vi "Test_StartMessageCycle_StopActor_OneOrMoreReceived.vi"(8 "error in (no error)":errorcluster, 11 "TestCase in":refnum<class "TestMessageCycle.lvclass">) -> (0 "error out":errorcluster, 3 "TestCase out":refnum<class "TestMessageCycle.lvclass">)   [LabVIEW 2017, in "TestMessageCycle.lvclass"]
uses:
  TestMessageCycle.lvclass
  Source/MessageCycle/MessageCycle.lvclass/MessageCycle.ctl
  <vilib>/ActorFramework/Message Enqueuer/Message Enqueuer.lvclass/Message Enqueuer.ctl
  <vilib>/ActorFramework/Message Enqueuer/Enqueue.vi
  Doubles/MessageCountsExecutions/MessageCountsExecutions.lvclass
  C:/Program Files (x86)/National Instruments/LabVIEW 2017/vi.lib/ActorFramework/Message/Message.lvclass
  Doubles/ActorCountsMessageCycles/ActorCountsMessageCycles.lvclass
  C:/Program Files (x86)/National Instruments/LabVIEW 2017/vi.lib/ActorFramework/Actor/Actor.lvclass
  Source/MessageCycle/MessageCycle.lvclass
  <vilib>/ActorFramework/Stop Msg/Stop Msg.lvclass
  Source/MessageCycle/Launch Deferred Timeout Notifier.vi
  <vilib>/ActorFramework/Message Priority Queue/Priority Enqueue.vi
  <vilib>/ActorFramework/Message/Message.lvclass
  <vilib>/ActorFramework/Actor/Actor.lvclass
panel:
  out "Messages Executed":u32
  out "Cyclic Messages Received":u32
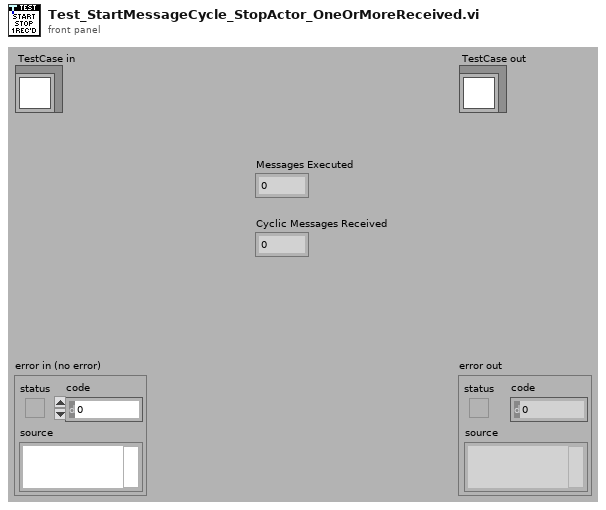
[diagram p1: front panel]
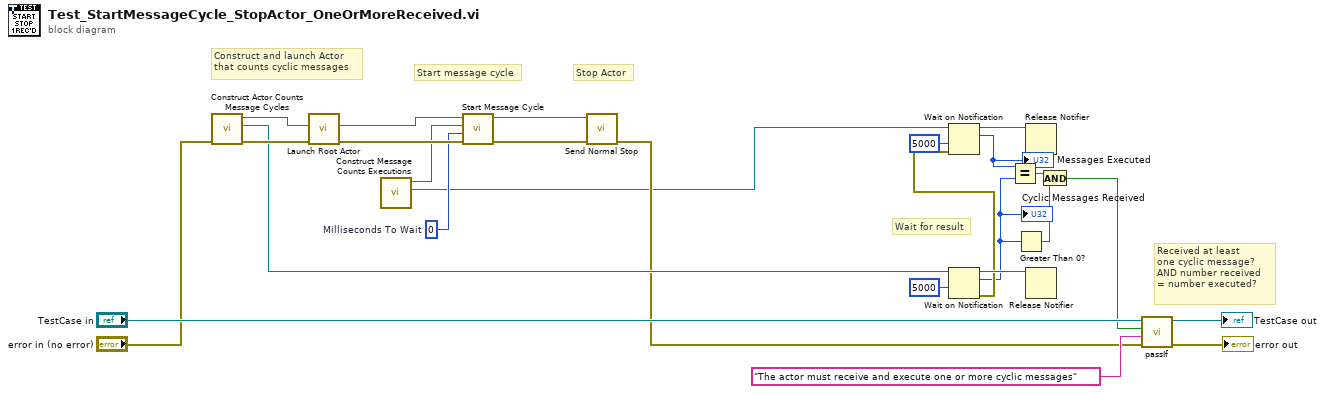
[diagram p0: block diagram]
diagram:
  w22 = 0  # Milliseconds To Wait
  # "Wait for result"
  # "Stop Actor"
  # "Start message cycle"
  # "Received at least\none cyclic message?\nAND number received\n= number executed?"
  # "Construct and launch Actor\nthat counts cyclic messages"
  n1 = call "Construct Actor Counts Message Cycles.vi"("error in (no error)"="error in (no error)") -> ("error out"=w15:errorcluster, "Final Count"=w14:refnum<notifier>, "ActorCountsMessageCycles"=w17:refnum<class "ActorCountsMessageCycles.lvclass">)  [unwired: 8 in]
  n2 = call <vilib>:"Launch Root Actor.vi"("error in (no error)"=w15, "Actor"=w17) -> ("error out"=w26:errorcluster, "Actor's Enqueuer"=w20:refnum<class "Message Enqueuer.lvclass">)  [unwired: 8 in]
  n3 = call "Construct Message Counts Executions.vi"() -> ("Message Executions"=w7:refnum<notifier>, "CyclicMessageCountsCycles out"=w8:refnum<class "MessageCountsExecutions.lvclass">)  [unwired: 9 in, 1 out]
  n4 = call "Start Message Cycle.vi"("error in (no error)"=w26, "Inter-Message Wait [ms] (0)"=w22, "Message"=w8, "Message Enqueuer"=w20) -> ("error out"=w21:errorcluster, "Message Enqueuer out"=w19:refnum<class "Message Enqueuer.lvclass">)  [unwired: 5 in, 1 out]
  n5 = call <vilib>:"Send Normal Stop.vi"("error in (no error)"=w21, "Message Enqueuer"=w19) -> ("error out"=w11:errorcluster)  [unwired: 9 in]
  n6 = Wait on Notification(notifier=w14, timeout in ms (-1)=5000) -> (notifier out=w12:refnum<notifier>, notification=w3:u32, error out=w6:errorcluster)  [unwired: 2 in, 1 out]
  "Cyclic Messages Received" <- w3
  n7 = Wait on Notification(notifier=w7, timeout in ms (-1)=5000, error in (no error)=w6) -> (notifier out=w10:refnum<notifier>, notification=w4:u32)  [unwired: 1 in, 2 out]
  "Messages Executed" <- w4
  n8 = Equal?(x=w4, y=w3) -> (x = y?=w2:bool)
  n9 = Greater Than 0?(x=w3) -> (x > 0?=w5:bool)
  n10 = Release Notifier(notifier=w10) -> ()  [unwired: 2 in, 3 out]
  n11 = Release Notifier(notifier=w12) -> ()  [unwired: 2 in, 3 out]
  n12 = And(x=w2, y=w5) -> (x .and. y?=w1:bool)
  n13 = call-dynamic "passIf.vi"("error in (no error)"=w11, "message (\"\")"="The actor must receive and execute one or more cyclic messages" ("message (\"\")"), "pass"=w1, "TestCase in"="TestCase in") -> ("error out"=→"error out":errorcluster, "TestCase out"=→"TestCase out":refnum<class "TestMessageCycle.lvclass">)  [unwired: 6 in]
